vi "ExpLogLoad.vi"   [LabVIEW 2019]
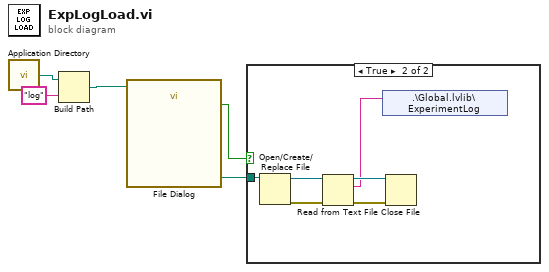
[diagram p0: block diagram]
diagram:
  n1 = call <vilib>:"Application Directory.vi"() -> ("Application Directory"=w5:path)
  n2 = Build Path(base path=w5, name or relative path="log") -> (appended path=w3:path)
  n3 = call "File Dialog"("start path"=w3) -> ("selected path"=w2:path, "exists"=w1:bool)  [unwired: 11 in, 2 out]
  n4 = case shown="True" w1 {
    tunnel: w2 -> [_ w11]
    frame False {
    }
    frame True {
      n5 = Open/Create/Replace File(file path (use dialog)=w11) -> (refnum out=w10:refnum<file>, error out=w9:errorcluster)  [unwired: 5 in, 1 out]
      n6 = Read from Text File(file (use dialog)=w10, error in=w9) -> (refnum out=w8:refnum<file>, text=w6:string, error out=w7:errorcluster)  [unwired: 2 in, 1 out]
      n7 = shared-variable ".\\Global.lvlib\\ExperimentLog"(w6) -> ()  [unwired: 1 in, 1 out]
      n8 = Close File(refnum=w8, error in=w7) -> ()  [unwired: 2 out]
    }
  }
